vi "SwissSPAD Live VIs Collection.vi"   [LabVIEW 2021]
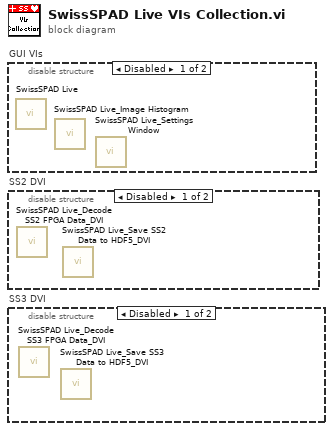
[diagram p0: block diagram]
diagram:
  n1 = disable-structure "GUI VIs" shown="Disabled" {
    frame Disabled {
      n2 = call "SwissSPAD Live.vi"() -> ()  [unwired: 12 in]
      n3 = call "SwissSPAD Live_Image Histogram.vi"() -> ()  [unwired: 12 in]
      n4 = call "SwissSPAD Live_Settings Window.vi"() -> ()  [unwired: 12 in]
    }
    frame Enabled {
    }
  }
  n5 = disable-structure "SS2 DVI" shown="Disabled" {
    frame Disabled {
      n6 = call "SwissSPAD Live_Decode SS2 FPGA Data_DVI.vi"() -> ()  [unwired: 12 in]
      n7 = call "SwissSPAD Live_Save SS2 Data to HDF5_DVI.vi"() -> ()  [unwired: 11 in, 1 out]
    }
    frame Enabled {
    }
  }
  n8 = disable-structure "SS3 DVI" shown="Disabled" {
    frame Disabled {
      n9 = call "SwissSPAD Live_Decode SS3 FPGA Data_DVI.vi"() -> ()  [unwired: 12 in]
      n10 = call "SwissSPAD Live_Save SS3 Data to HDF5_DVI.vi"() -> ()  [unwired: 11 in, 1 out]
    }
    frame Enabled {
    }
  }
